vi "PathPlanner_Cmd_AutoHolonomicExecute.vi"(5 "PathPlanner_Cmd_FollowHolConfig":T17={"HOLONOMIC_CTRL_PACK_TUNING"={"X PID Tuning"={"Kp"=0.0, "Ki"=0.0, "Kd"=0.0, "MaximumIntegral"=9.9e+30, "MinimumIntegral"=-9.9e+30, "IntegralZone"=9.9e+30}, "Y PID Tuning"={"Kp"=0.0, "Ki"=0.0, "Kd"=0.0, "MaximumIntegral"=9.9e+30, "MinimumIntegral"=-9.9e+30, "IntegralZone"=9.9e+30}, "thetaProfiledPID_CTRL"={"Controller"={"Kp"=0.0, "Ki"=0.0, "Kd"=0.0, "Period"=0.0, "Max_Integral"=1.0, "Min_Integral"=-1.0, "Max_Input"=0.0, "Min_Input"=0.0, "Continuous"=FALSE, "PositionError"=0.0, "VelocityError"=0.0, "PrevError"=0.0, "Total_Integral"=0.0, "PositionTolerance"=0.05, "VelocityTolerance"=9.99e+35, "SetPoint"=0.0, "Kf"=0.0, "Prev_Deriv"=0.0, "Prev_Deriv 2"=0.0, "DerivativeFilter"=FALSE, "Min_Output"=-9.99e+35, "Max_Output"=9.9e+35, "Prev_F_P"=0.0, "Prev_F_P_2"=0.0, "AntiWindupActive"=FALSE, "Measurement"=0.0, "IntegralZone"=9.9e+30}, "Goal"={"Position"=0.0, "Velocity"=0.0}, "Setpoint"={"Position"=0.0, "Velocity"=0.0}, "Constraint"={"MaxVelocity"=0.0, "MaxAcceleration"=0.0}}}, "Max Wheel Speed M/S"=0.0, "Tolerance SI"={"TRANSLATION"={"X"=0.04, "Y"=0.04}, "ROTATION"={"VALUE"=0.034906585039887, "COS"=0.999390827019096, "SIN"=0.034899496702501}}, "Drive Base Radius M"=0.0, "ControlPastEnd_Sec"=3.0, "Period_Sec"=0.02, "Trigger Events"=TRUE} {"Tolerance SI"."ROTATION"."SIN" format="%13.4f"; "Tolerance SI"."ROTATION"."COS" format="%13.4f"; "Tolerance SI"."ROTATION"."VALUE" format="%13.4f"; "Tolerance SI"."TRANSLATION"."Y" format="%14.3f"; "Tolerance SI"."TRANSLATION"."X" format="%14.3f"; "HOLONOMIC_CTRL_PACK_TUNING"."thetaProfiledPID_CTRL"."Constraint"."MaxAcceleration" format="%16_6e"; "HOLONOMIC_CTRL_PACK_TUNING"."thetaProfiledPID_CTRL"."Constraint"."MaxVelocity" format="%16_6e"; "HOLONOMIC_CTRL_PACK_TUNING"."thetaProfiledPID_CTRL"."Setpoint"."Velocity" format="%16_6e"; "HOLONOMIC_CTRL_PACK_TUNING"."thetaProfiledPID_CTRL"."Setpoint"."Position" format="%16_6e"; "HOLONOMIC_CTRL_PACK_TUNING"."thetaProfiledPID_CTRL"."Goal"."Velocity" format="%16_6e"; "HOLONOMIC_CTRL_PACK_TUNING"."thetaProfiledPID_CTRL"."Goal"."Position" format="%16_6e"; "HOLONOMIC_CTRL_PACK_TUNING"."thetaProfiledPID_CTRL"."Controller"."IntegralZone" format="%16_6e"; "HOLONOMIC_CTRL_PACK_TUNING"."thetaProfiledPID_CTRL"."Controller"."Measurement" format="%16_6e"; "HOLONOMIC_CTRL_PACK_TUNING"."thetaProfiledPID_CTRL"."Controller"."Prev_F_P_2" format="%16_6e"; "HOLONOMIC_CTRL_PACK_TUNING"."thetaProfiledPID_CTRL"."Controller"."Prev_F_P" format="%16_6e"; "HOLONOMIC_CTRL_PACK_TUNING"."thetaProfiledPID_CTRL"."Controller"."Max_Output" format="%16_6e"; "HOLONOMIC_CTRL_PACK_TUNING"."thetaProfiledPID_CTRL"."Controller"."Min_Output" format="%16_6e"; "HOLONOMIC_CTRL_PACK_TUNING"."thetaProfiledPID_CTRL"."Controller"."Prev_Deriv 2" format="%16_6e"; "HOLONOMIC_CTRL_PACK_TUNING"."thetaProfiledPID_CTRL"."Controller"."Prev_Deriv" format="%16_6e"; "HOLONOMIC_CTRL_PACK_TUNING"."thetaProfiledPID_CTRL"."Controller"."Kf" format="%16_6e"; "HOLONOMIC_CTRL_PACK_TUNING"."thetaProfiledPID_CTRL"."Controller"."SetPoint" format="%16_6e"; "HOLONOMIC_CTRL_PACK_TUNING"."thetaProfiledPID_CTRL"."Controller"."VelocityTolerance" format="%16_6e"; "HOLONOMIC_CTRL_PACK_TUNING"."thetaProfiledPID_CTRL"."Controller"."PositionTolerance" format="%16_6e"; "HOLONOMIC_CTRL_PACK_TUNING"."thetaProfiledPID_CTRL"."Controller"."Total_Integral" format="%16_6e"; "HOLONOMIC_CTRL_PACK_TUNING"."thetaProfiledPID_CTRL"."Controller"."PrevError" format="%16_6e"; "HOLONOMIC_CTRL_PACK_TUNING"."thetaProfiledPID_CTRL"."Controller"."VelocityError" format="%16_6e"; "HOLONOMIC_CTRL_PACK_TUNING"."thetaProfiledPID_CTRL"."Controller"."PositionError" format="%16_6e"; "HOLONOMIC_CTRL_PACK_TUNING"."thetaProfiledPID_CTRL"."Controller"."Min_Input" format="%16_6e"; "HOLONOMIC_CTRL_PACK_TUNING"."thetaProfiledPID_CTRL"."Controller"."Max_Input" format="%16_6e"; "HOLONOMIC_CTRL_PACK_TUNING"."thetaProfiledPID_CTRL"."Controller"."Min_Integral" format="%16_6e"; "HOLONOMIC_CTRL_PACK_TUNING"."thetaProfiledPID_CTRL"."Controller"."Max_Integral" format="%16_6e"; "HOLONOMIC_CTRL_PACK_TUNING"."thetaProfiledPID_CTRL"."Controller"."Period" format="%16_6e"; "HOLONOMIC_CTRL_PACK_TUNING"."thetaProfiledPID_CTRL"."Controller"."Kd" format="%16_6e"; "HOLONOMIC_CTRL_PACK_TUNING"."thetaProfiledPID_CTRL"."Controller"."Ki" format="%16_6e"; "HOLONOMIC_CTRL_PACK_TUNING"."thetaProfiledPID_CTRL"."Controller"."Kp" format="%16_6e"}, 6 "PassthroughTime_SEC":dbl=-1.0, 7 "PathPlanner_Cmd_AutoConfig":T2 {"Paths"."IdealStartingState"."Rotation"."SIN" format="%13.4f"; "Paths"."IdealStartingState"."Rotation"."COS" format="%13.4f"; "Paths"."IdealStartingState"."Rotation"."VALUE" format="%13.4f"; "Paths"."PointTowardsZones"."TargetPosition"."Y" format="%14.3f"; "Paths"."PointTowardsZones"."TargetPosition"."X" format="%14.3f"; "Paths"."PointTowardsZones"."RotationOffset"."SIN" format="%13.4f"; "Paths"."PointTowardsZones"."RotationOffset"."COS" format="%13.4f"; "Paths"."PointTowardsZones"."RotationOffset"."VALUE" format="%13.4f"; "Paths"."Waypoints"."nextControl"."Y" format="%14.3f"; "Paths"."Waypoints"."nextControl"."X" format="%14.3f"; "Paths"."Waypoints"."anchor"."Y" format="%14.3f"; "Paths"."Waypoints"."anchor"."X" format="%14.3f"; "Paths"."Waypoints"."prevControl"."Y" format="%14.3f"; "Paths"."Waypoints"."prevControl"."X" format="%14.3f"; "Paths"."AllPoints"."RotationTarget"."rotation"."SIN" format="%13.4f"; "Paths"."AllPoints"."RotationTarget"."rotation"."COS" format="%13.4f"; "Paths"."AllPoints"."RotationTarget"."rotation"."VALUE" format="%13.4f"; "Paths"."AllPoints"."Position"."Y" format="%14.3f"; "Paths"."AllPoints"."Position"."X" format="%14.3f"; "Paths"."GoalEndState"."Rotation"."SIN" format="%13.4f"; "Paths"."GoalEndState"."Rotation"."COS" format="%13.4f"; "Paths"."GoalEndState"."Rotation"."VALUE" format="%13.4f"; "Paths"."RotationTargets"."rotation"."SIN" format="%13.4f"; "Paths"."RotationTargets"."rotation"."COS" format="%13.4f"; "Paths"."RotationTargets"."rotation"."VALUE" format="%13.4f"}, 8 "Enabled":bool=TRUE, 9 "Reset":bool, 10 "CurrentChassisSpeeds":T1 {"vOmega" format="%10.3f"; "vY" format="%10.3f"; "vX" format="%10.3f"}, 11 "Current Pose SI":T24={"TRANSLATION"={"X"=0.0, "Y"=0.0}, "ROTATION"={"VALUE"=0.0, "COS"=1.0, "SIN"=0.0}} {"ROTATION"."SIN" format="%13.4f"; "ROTATION"."COS" format="%13.4f"; "ROTATION"."VALUE" format="%13.4f"; "TRANSLATION"."Y" format="%14.3f"; "TRANSLATION"."X" format="%14.3f"}) -> (0 "Position Error M":dbl, 1 "Complete":bool, 2 "At Reference":bool, 3 "calcChassisSpeed":T1 {"vOmega" format="%10.3f"; "vY" format="%10.3f"; "vX" format="%10.3f"})   [LabVIEW 2019, in "PathPlanner24.lvlib"]
doc: "DOCUMENTATION IS NOT COMPLETE.\n \nCalculates the next output of the path following controller for holonomic drive robots. This wraps a Holonomic Drive Control function with the particulars needed to follow a PathPlanner trajectory.\n\nInputs:\n - PathPlanner_Holonomic_Ctrl_Pack_Tuning - cluster - The tuning paraameters for the holonomic drive controller. These are static. They should not be changed after the first call to this function.\n - CurrentPoseSi - pose2d - The current pose calculated by odometry or pose estimation. The pose can be absolute or relative depending on what type of trajectory is being followed.\n - PathPlannerState - cluster - The path palnner trajectory state containing the desired position and velocities of the robot.\n - Reset - boolean - When TRUE the holonomic drive controller is reset. This should be set to TRUE for the first execution of a trajectory.\n - Enabled - boolean - When TRUE, closed loop control is enabled. (Optional. Default: TRUE)\n - Period - double - The loop period in seconds for this controller. (Optional. Default: 0.020)\n\nOutputs:\n - CalcChassisSpeed - cluster - The desired chassis speed in SI units.\n - AtReference - boolean - TRUE if the robots position is within the defined tolerance.\n - PositionError - pose2d - Position error in SI units. How far the robot is away from the desired trajectory position.\n - out_Holonomic_Drive_Ctrl - THe current holonomic drive controller data cluster. This is mainly for diagnostic purposes."
uses:
  PathPlanner24.lvlib
  <vilib>/Rock Robotics/WPI/ThirdParty/JAS_Junk/TrajLib/Trajectory_Library.lvlib
  <vilib>/Rock Robotics/WPI/ThirdParty/JAS_Junk/TrajLib/TypeDef/CHASSIS_SPEEDS.ctl
  <vilib>/Rock Robotics/WPI/ThirdParty/JAS_Junk/TrajLib/TypeDef/TRANSLATION2D.ctl
  <vilib>/Rock Robotics/WPI/ThirdParty/JAS_Junk/TrajLib/TypeDef/ROTATION2D.ctl
  <vilib>/Rock Robotics/WPI/ThirdParty/JAS_Junk/TrajLib/TypeDef/POSE2D.ctl
  <vilib>/Rock Robotics/WPI/ThirdParty/JAS_Junk/TrajLib/TypeDef/PID_TUNING.ctl
  <vilib>/Rock Robotics/WPI/ThirdParty/JAS_Junk/TrajLib/TypeDef/PID_CONTROLLER.ctl
  <vilib>/Rock Robotics/WPI/ThirdParty/JAS_Junk/TrajLib/TypeDef/TRAPEZOID_PROFILE_STATE.ctl
  <vilib>/Rock Robotics/WPI/ThirdParty/JAS_Junk/TrajLib/TypeDef/TRAPEZOID_PROFILE_CONSTRAINT.ctl
  <vilib>/Rock Robotics/WPI/ThirdParty/JAS_Junk/TrajLib/TypeDef/PROFILED_PID_CONTROLLER.ctl
  <vilib>/Rock Robotics/WPI/ThirdParty/JAS_Junk/TrajLib/TypeDef/HOLONOMIC_PACK_TUNING.ctl
  TypeDef/PathPlannerRotationTarget.ctl
  TypeDef/PathPlannerPathConstraints.ctl
  TypeDef/PathPlannerConstraintsZone.ctl
  ENum/PathPlanner_CommandUtilType_ENUM.ctl
  TypeDef/PathPlannerCommandUtil.ctl
  TypeDef/PathPlannerEventMarker.ctl
  TypeDef/PathPlannerGoalEndState.ctl
  TypeDef/PathPlannerPathPoint.ctl
  TypeDef/PathPlannerPath.ctl
  TypeDef/PathPlannerCmdFollowHolConfig.ctl
  TypeDef/PathPlannerWaypoint.ctl
  TypeDef/PathPlannerPointTowardsZone.ctl
  TypeDef/PathPlannerIdealStartingState.ctl
  TypeDef/PathPlannerCmdPathPlannerAutoConfig.ctl
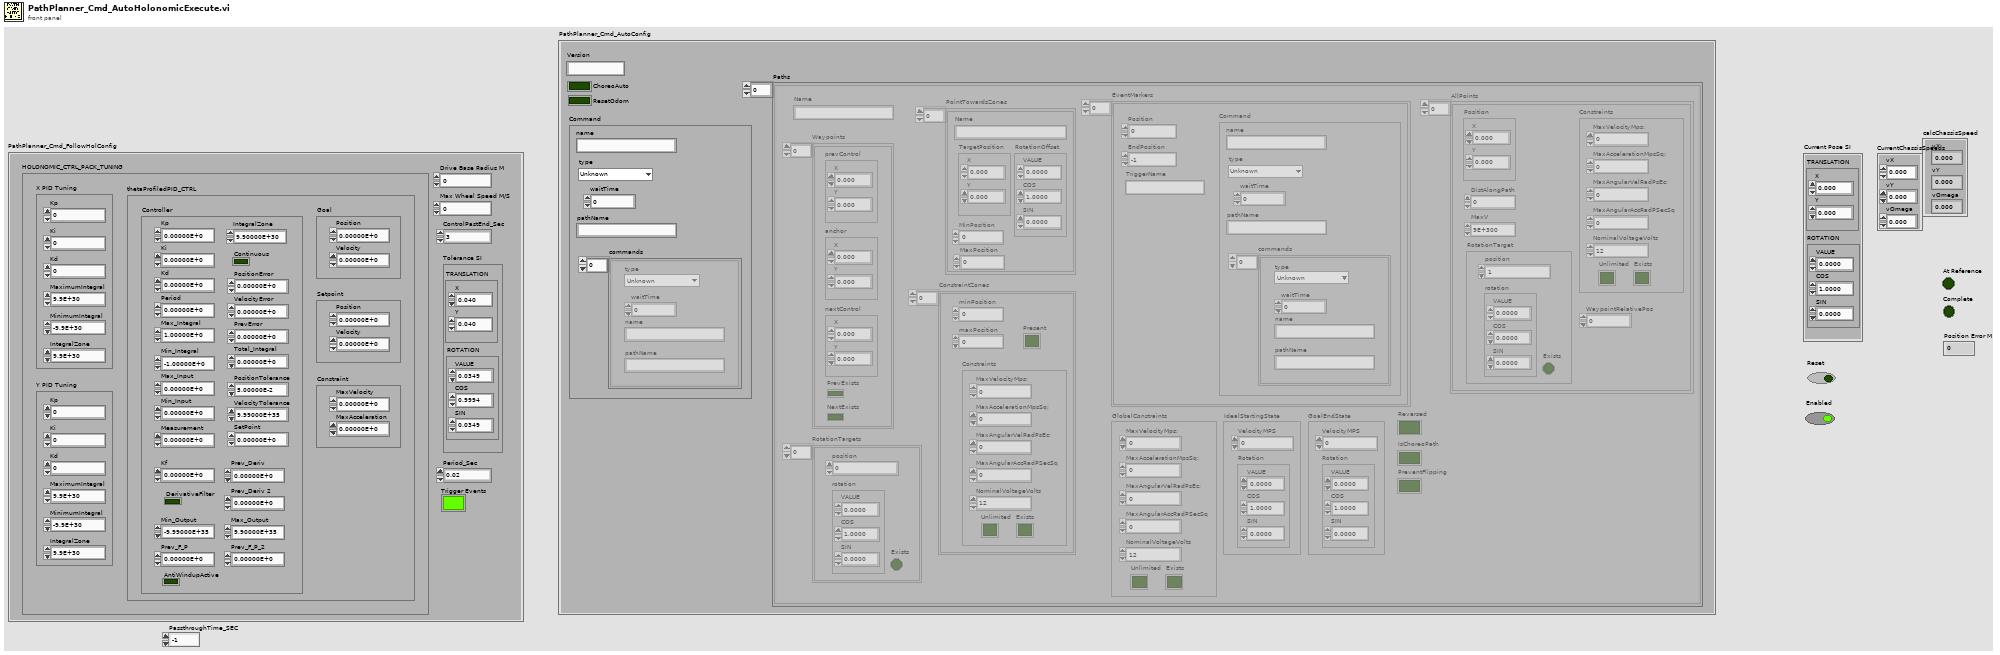
[diagram p1: front panel]
types:
  T1 = typedef "Trajectory_Library.lvlib/CHASSIS_SPEEDS.ctl" = cluster{"vX":dbl, "vY":dbl, "vOmega":dbl}
  T2 = typedef "PathPlanner24.lvlib/PathPlannerCmdPathPlannerAutoConfig.ctl" = cluster{"Command":T3, "ChoreoAuto":bool, "Version":string, "ResetOdom":bool, "Paths":T5[]}
  T3 = typedef "PathPlanner24.lvlib/PathPlannerCommandUtil.ctl" = cluster{"waitTime":dbl, "name":string, "pathName":string, "commands":cluster{"type":T4, "waitTime":dbl, "name":string, "pathName":string}[], "type":T4}
  T4 = typedef "PathPlanner24.lvlib/PathPlanner_CommandUtilType_ENUM.ctl" = enum16{"Unknown", "Wait", "Named", "Path", "Sequential", "Parallel", "Race", "Deadline"}
  T5 = typedef "PathPlanner24.lvlib/PathPlannerPath.ctl" = cluster{"Reversed":bool, "RotationTargets":T6[], "ConstraintZones":T8[], "EventMarkers":T10[], "GlobalConstraints":T9, "GoalEndState":T11, "AllPoints":T12[], "Name":string, "Waypoints":T14[], "PointTowardsZones":T15[], "IdealStartingState":T16, "IsChoreoPath":bool, "PreventFlipping":bool}
  T6 = typedef "PathPlanner24.lvlib/PathPlannerRotationTarget.ctl" = cluster{"position":dbl, "rotation":T7, "Exists":bool}
  T7 = typedef "Trajectory_Library.lvlib/ROTATION2D.ctl" = cluster{"VALUE":dbl, "COS":dbl, "SIN":dbl}
  T8 = typedef "PathPlanner24.lvlib/PathPlannerConstraintsZone.ctl" = cluster{"minPosition":dbl, "maxPosition":dbl, "Constraints":T9, "Present":bool}
  T9 = typedef "PathPlanner24.lvlib/PathPlannerPathConstraints.ctl" = cluster{"MaxVelocityMps;":dbl, "MaxAccelerationMpsSq;":dbl, "MaxAngularVelRadPsEc;":dbl, "MaxAngularAccRadPSecSq":dbl, "Exists":bool, "Unlimited":bool, "NominalVoltageVolts":dbl}
  T10 = typedef "PathPlanner24.lvlib/PathPlannerEventMarker.ctl" = cluster{"Position":dbl, "Command":T3, "TriggerName":string, "EndPosition":dbl}
  T11 = typedef "PathPlanner24.lvlib/PathPlannerGoalEndState.ctl" = cluster{"VelocityMPS":dbl, "Rotation":T7}
  T12 = typedef "PathPlanner24.lvlib/PathPlannerPathPoint.ctl" = cluster{"Position":T13, "DistAlongPath":dbl, "MaxV":dbl, "Constraints":T9, "RotationTarget":T6, "WaypointRelativePos":dbl}
  T13 = typedef "Trajectory_Library.lvlib/TRANSLATION2D.ctl" = cluster{"X":dbl, "Y":dbl}
  T14 = typedef "PathPlanner24.lvlib/PathPlannerWaypoint.ctl" = cluster{"prevControl":T13, "anchor":T13, "nextControl":T13, "PrevExists":bool, "NextExists":bool}
  T15 = typedef "PathPlanner24.lvlib/PathPlannerPointTowardsZone.ctl" = cluster{"RotationOffset":T7, "Name":string, "TargetPosition":T13, "MinPosition":dbl, "MaxPosition":dbl}
  T16 = typedef "PathPlanner24.lvlib/PathPlannerIdealStartingState.ctl" = cluster{"VelocityMPS":dbl, "Rotation":T7}
  T17 = typedef "PathPlanner24.lvlib/PathPlannerCmdFollowHolConfig.ctl" = cluster{"HOLONOMIC_CTRL_PACK_TUNING":T18, "Max Wheel Speed M/S":dbl, "Tolerance SI":T24, "Drive Base Radius M":dbl, "ControlPastEnd_Sec":dbl, "Period_Sec":dbl, "Trigger Events":bool}
  T18 = typedef "Trajectory_Library.lvlib/HOLONOMIC_PACK_TUNING.ctl" = cluster{"X PID Tuning":T19, "Y PID Tuning":T19, "thetaProfiledPID_CTRL":T20}
  T19 = typedef "Trajectory_Library.lvlib/PID_TUNING.ctl" = cluster{"Kp":dbl, "Ki":dbl, "Kd":dbl, "MaximumIntegral":dbl, "MinimumIntegral":dbl, "IntegralZone":dbl}
  T20 = typedef "Trajectory_Library.lvlib/PROFILED_PID_CONTROLLER.ctl" = cluster{"Controller":T21, "Goal":T22, "Setpoint":T22, "Constraint":T23}
  T21 = typedef "Trajectory_Library.lvlib/PID_CONTROLLER.ctl" = cluster{"Kp":dbl, "Ki":dbl, "Kd":dbl, "Period":dbl, "Max_Integral":dbl, "Min_Integral":dbl, "Max_Input":dbl, "Min_Input":dbl, "Continuous":bool, "PositionError":dbl, "VelocityError":dbl, "PrevError":dbl, "Total_Integral":dbl, "PositionTolerance":dbl, "VelocityTolerance":dbl, "SetPoint":dbl, "Kf":dbl, "Prev_Deriv":dbl, "Prev_Deriv 2":dbl, "DerivativeFilter":bool, "Min_Output":dbl, "Max_Output":dbl, "Prev_F_P":dbl, "Prev_F_P_2":dbl, "AntiWindupActive":bool, "Measurement":dbl, "IntegralZone":dbl}
  T22 = typedef "Trajectory_Library.lvlib/TRAPEZOID_PROFILE_STATE.ctl" = cluster{"Position":dbl, "Velocity":dbl}
  T23 = typedef "Trajectory_Library.lvlib/TRAPEZOID_PROFILE_CONSTRAINT.ctl" = cluster{"MaxVelocity":dbl, "MaxAcceleration":dbl}
  T24 = typedef "Trajectory_Library.lvlib/POSE2D.ctl" = cluster{"TRANSLATION":T13, "ROTATION":T7}
  T25 = typedef "Trajectory_Library.lvlib/TIMER.ctl" = cluster{"StartTime":dbl, "Accumulated TIme":dbl, "Running":bool, "semaphore":T26}
  T26 = typedef "Semaphore RefNum" = refnum<k1>
  T27 = cluster{"type":T4, "waitTime":dbl, "name":string, "pathName":string}[]
  T28 = cluster{"type":T4, "waitTime":dbl, "name":string, "pathName":string}
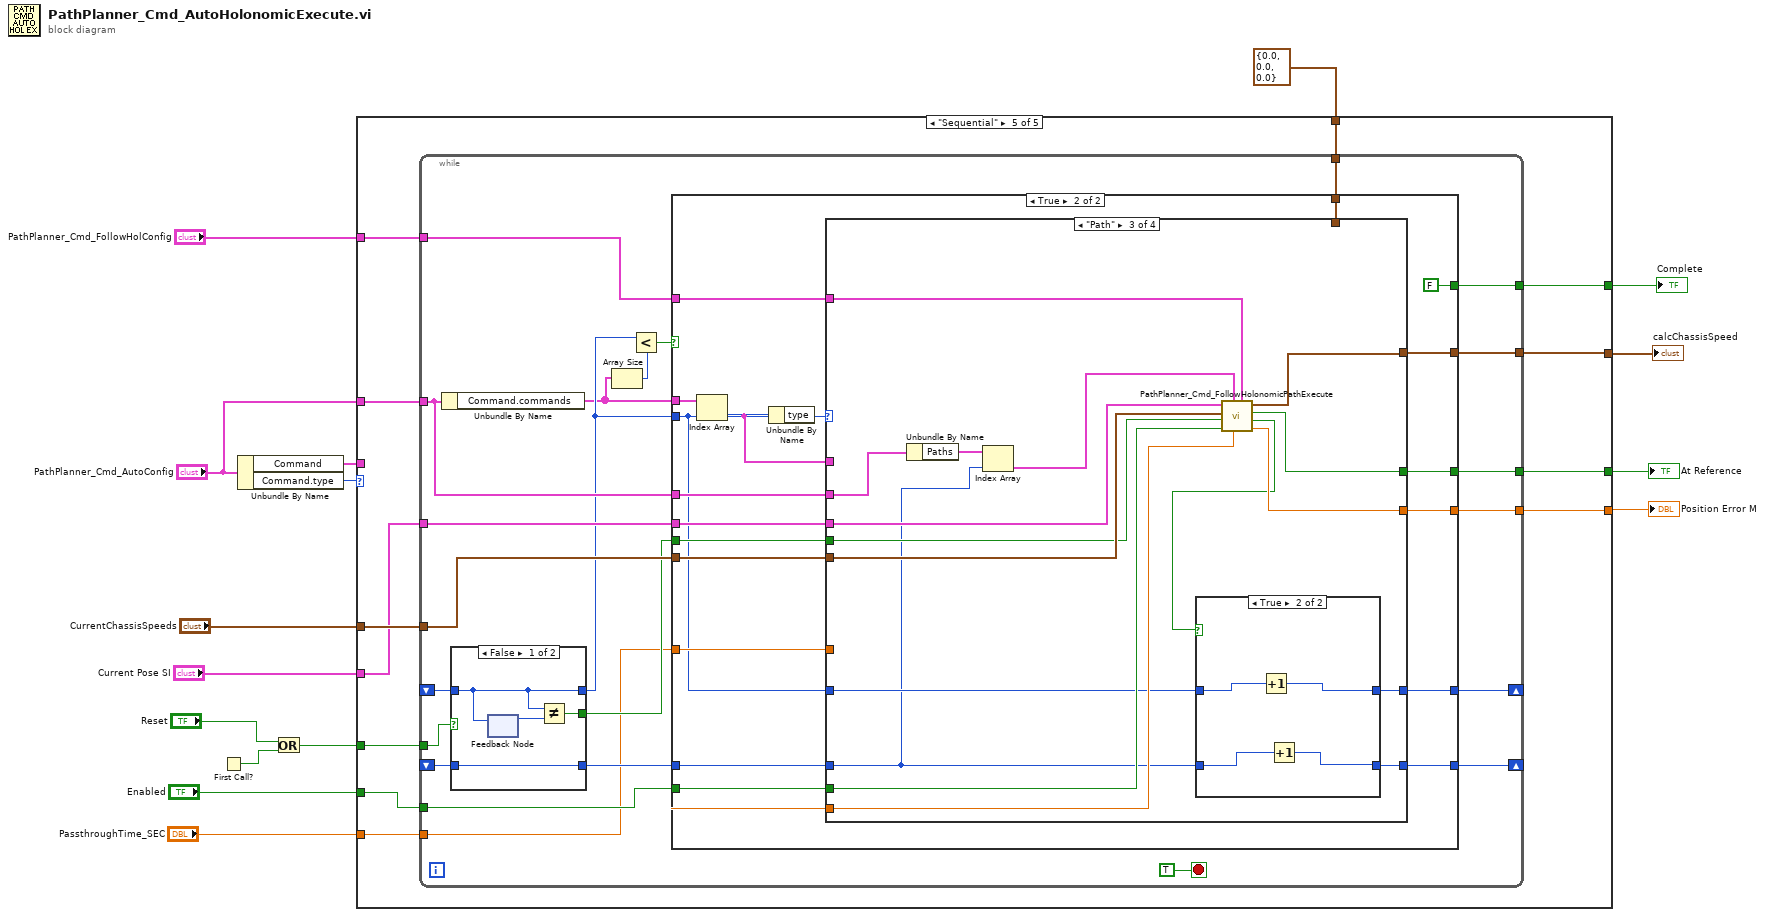
[diagram p0: block diagram]
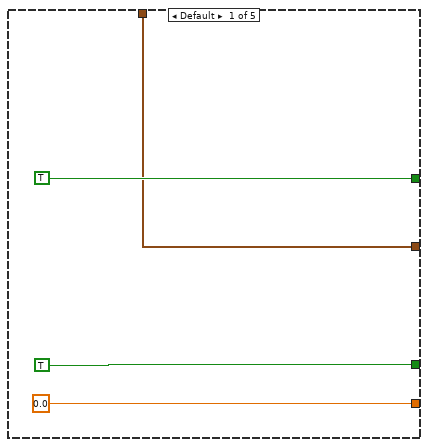
[diagram p2: hidden frame]
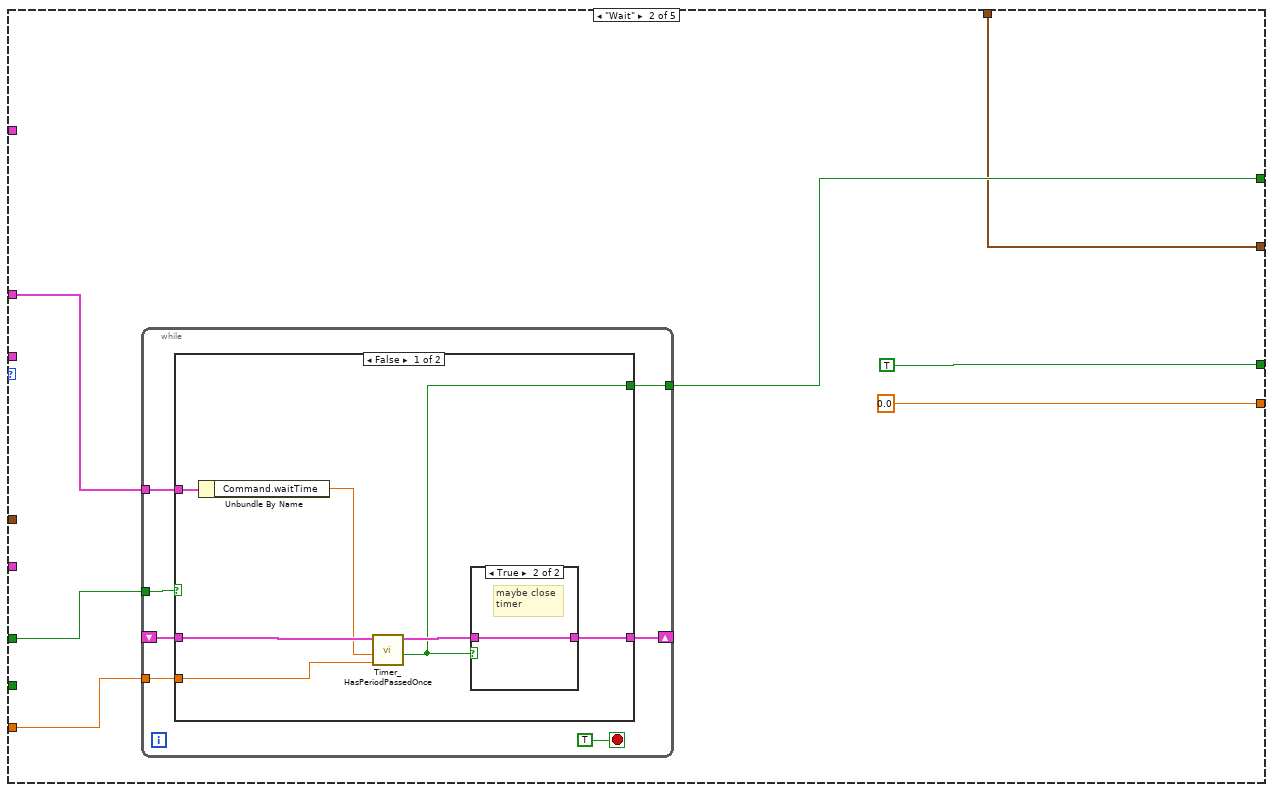
[diagram p3: hidden frame]
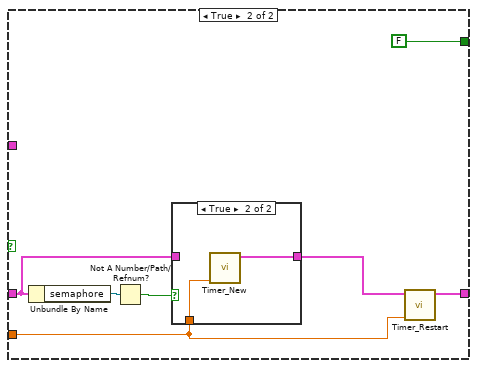
[diagram p5: hidden frame]
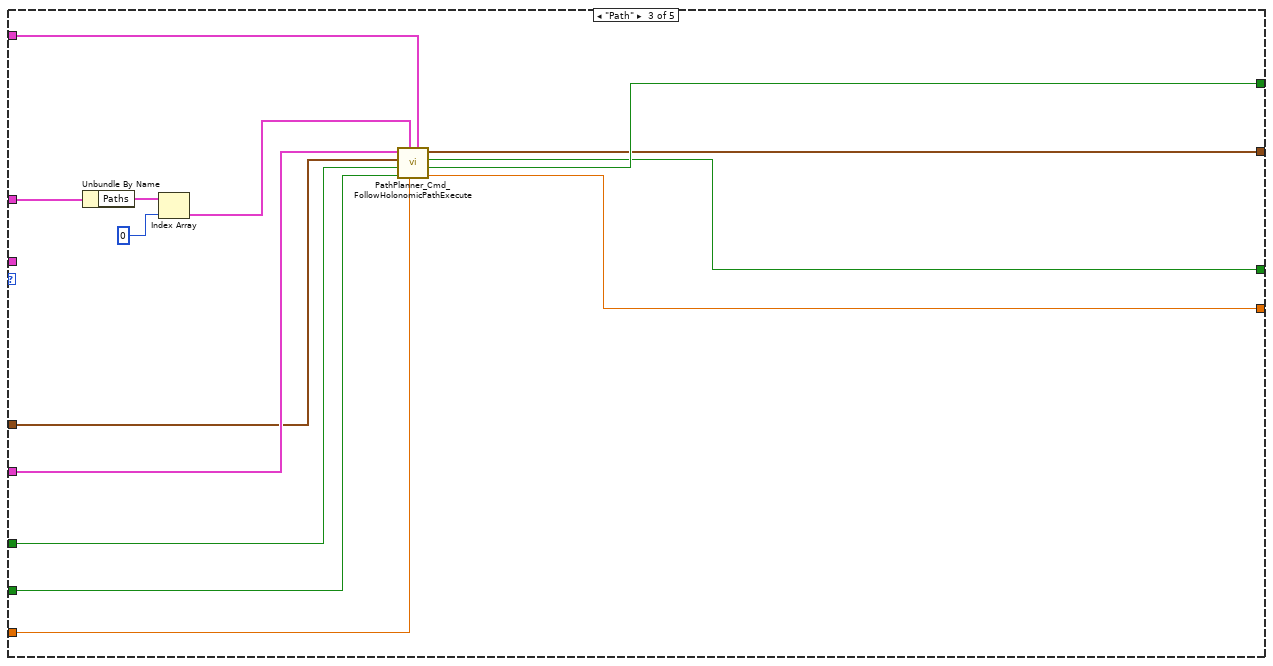
[diagram p7: hidden frame]
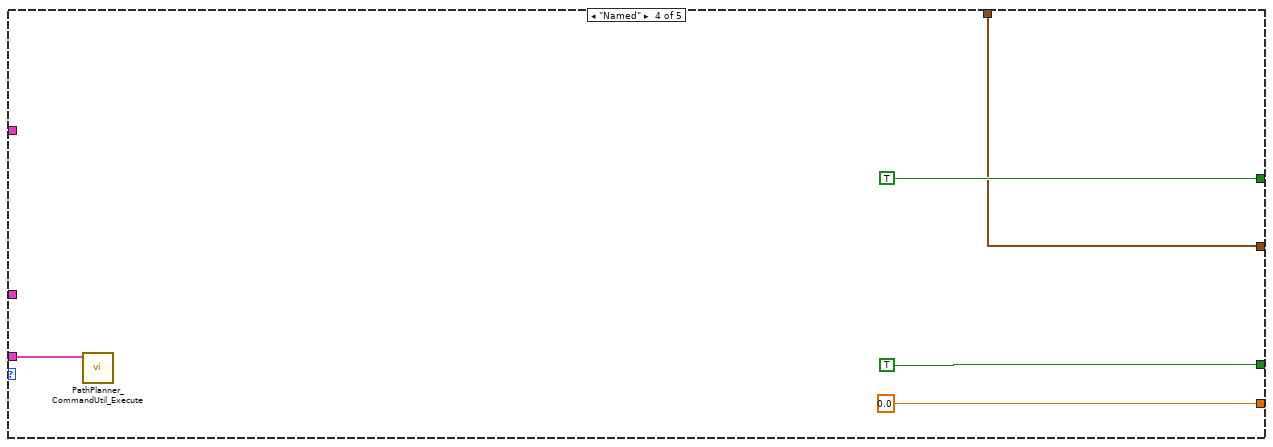
[diagram p8: hidden frame]
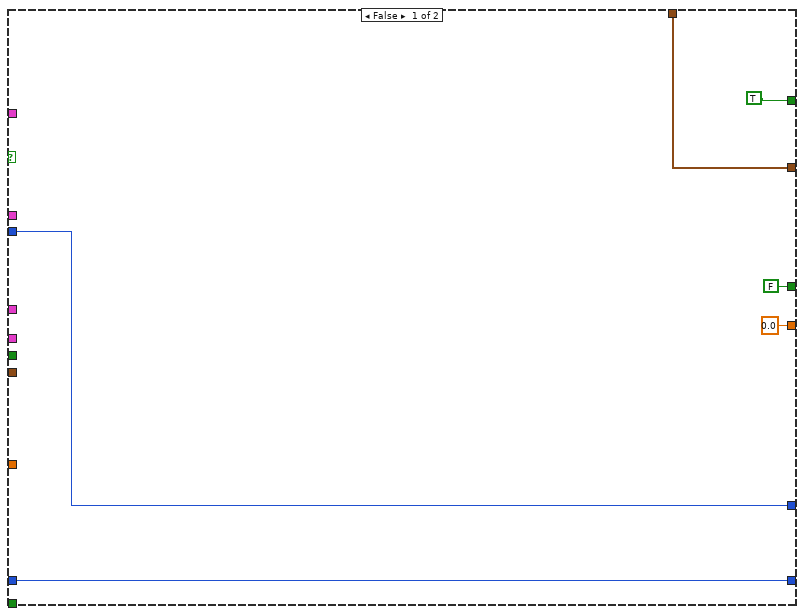
[diagram p9: hidden frame]
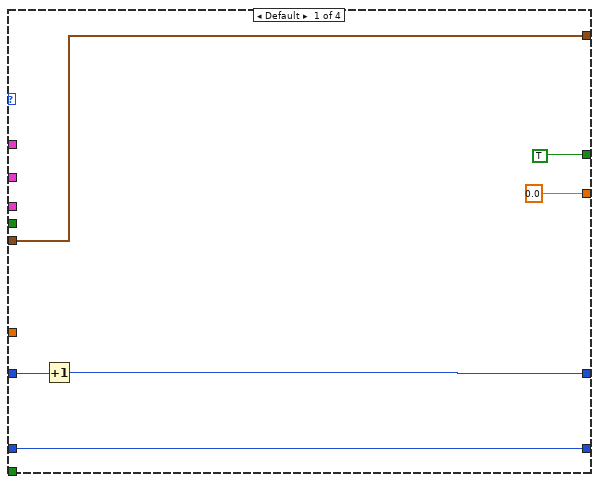
[diagram p10: hidden frame]
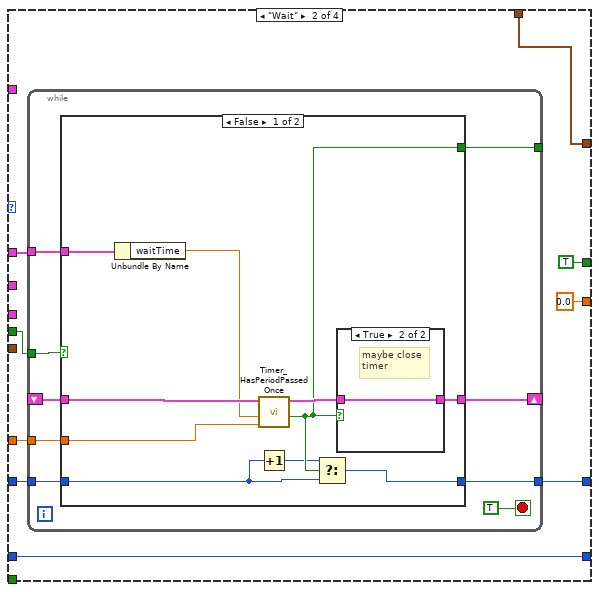
[diagram p11: hidden frame]
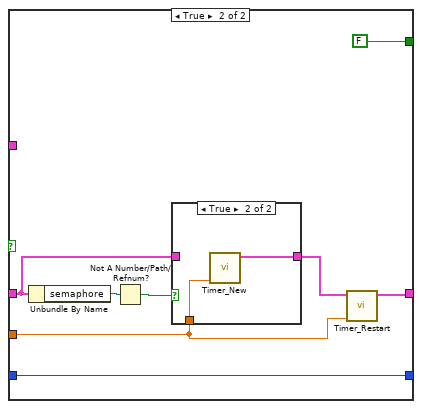
[diagram p13: hidden frame]
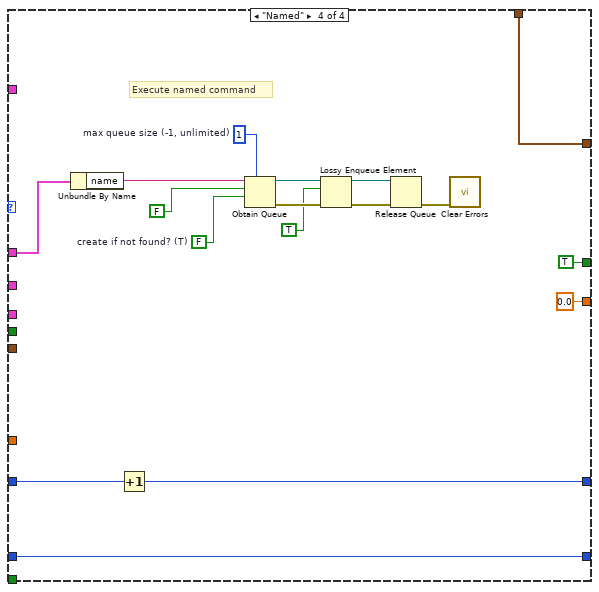
[diagram p16: hidden frame]
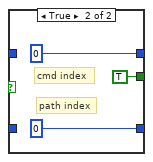
[diagram p17: hidden frame]
diagram:
  n1 = First Call?() -> (First Call?: T/F=w15:bool)
  n2 = Unbundle By Name("PathPlanner_Cmd_AutoConfig") -> ("Command"=w13:T3, "Command.type"=w14:T4)
  n3 = Or(x="Reset", y=w15) -> (x .or. y?=w8:bool)
  n4 = case shown="\"Sequential\"" w14 {
    tunnel: w13 -> [_ _ _ w72 _]
    tunnel: "PathPlanner_Cmd_AutoConfig" -> [_ w25 w67 _ w83]
    tunnel: "PathPlanner_Cmd_FollowHolConfig" -> [_ _ w63 _ w76]
    tunnel: "Current Pose SI" -> [_ _ w62 _ w75]
    tunnel: "CurrentChassisSpeeds" -> [_ _ w61 _ w82]
    tunnel: w8 -> [_ w27 w60 _ w84]
    tunnel: "Enabled" -> [_ _ w59 _ w74]
    tunnel: "PassthroughTime_SEC" -> [_ w26 w58 _ w78]
    tunnel: [0.0 ("Position Error M") 0.0 ("Position Error M") w57 0.0 ("Position Error M") w79] -> w5
    tunnel: [TRUE ("Complete") w24 w56 TRUE ("Complete") w73] -> w4
    tunnel: [TRUE ("At Reference") TRUE ("At Reference") w55 TRUE ("At Reference") w80] -> w3
    tunnel: [w17 w21 w54 w68 w81] -> w2
    tunnel: T1 {"vX"=0.0, "vY"=0.0, "vOmega"=0.0} ("CurrentChassisSpeeds") -> [w17 w21 _ w68 w77]
    frame Default {
    }
    frame "Wait" {
      n5 = while {
        tunnel: w27 -> [w34]
        tunnel: w26 -> [w33]
        shift-right: [w32] -> _
        shift-left: _ -> [w31]
        tunnel: w25 -> [w30]
        tunnel: [w28] -> w24
        stop <- TRUE stop-if-true
        n6 = case shown="False" w34 {
          tunnel: w33 -> [w40 w49]
          tunnel: [w36 w48] -> w32
          tunnel: w31 -> [w41 w44]
          tunnel: w30 -> [w39 _]
          tunnel: [w35 FALSE ("Expired")] -> w28
          frame False {
            n7 = Unbundle By Name(w39) -> ("Command.waitTime"=w38:dbl)
            n8 = call <vilib>:"Timer_HasPeriodPassedOnce.vi"("Pass_Through_Time"=w40, "Period"=w38, "in Timer"=w41) -> ("Expired"=w35:bool, "out Timer"=w37:T25)  [unwired: 6 in, 1 out]
            n9 = case shown="True" w35 {
              tunnel: w37 -> [w42 w43]
              tunnel: [w42 w43] -> w36
              frame False {
              }
              frame True {
                # "maybe close\ntimer"
              }
            }
          }
          frame True {
            n10 = Unbundle By Name(w44) -> ("semaphore"=w45:T26)
            n11 = Not A Number/Path/Refnum?(number/path/refnum=w45) -> (NaN/Path/Refnum?=w46:bool)
            n12 = case shown="True" w46 {
              tunnel: [w51 w53] -> w50
              tunnel: w49 -> [_ w52]
              tunnel: w44 -> [w51 _]
              frame False {
              }
              frame True {
                n13 = call <vilib>:"Timer_New.vi"("Pass_Through_Time"=w52) -> ("TIMER"=w53:T25)  [unwired: 10 in]
              }
            }
            n14 = call <vilib>:"Timer_Restart.vi"("Pass_Through_Time"=w49, "in Timer"=w50) -> ("out Timer"=w48:T25)  [unwired: 9 in]
          }
        }
      }
    }
    frame "Path" {
      n15 = Unbundle By Name(w67) -> ("Paths"=w66:T5[])
      n16 = Index Array(array=w66, index=0) -> (element=w64:T5)
      n17 = call "PathPlanner_Cmd_FollowHolonomicPathExecute.vi"("PathPlanner_Cmd_FollowHolConfig"=w63, "PassthroughTime_SEC"=w58, "PathPlannerPath"=w64, "Enabled"=w59, "Reset"=w60, "CurrentChassisSpeeds"=w61, "Current Pose SI"=w62) -> ("Position Error M"=w57:dbl, "Complete"=w56:bool, "At Reference"=w55:bool, "calcChassisSpeed"=w54:T1)  [unwired: 1 out]
    }
    frame "Named" {
      n18 = call "PathPlanner_CommandUtil_Execute.vi"("Command"=w72) -> ()  [unwired: 11 in]
    }
    frame "Sequential" {
      n19 = while {
        tunnel: w84 -> [w102]
        tunnel: w83 -> [w97]
        tunnel: w82 -> [w106]
        tunnel: [w105] -> w81
        tunnel: [w104] -> w80
        tunnel: [w103] -> w79
        tunnel: w78 -> [w92]
        shift-right: [w91] -> _
        shift-left: _ -> [w101]
        shift-right: [w90] -> _
        shift-left: _ -> [w100]
        tunnel: w77 -> [w98]
        tunnel: w76 -> [w95]
        tunnel: w75 -> [w94]
        tunnel: w74 -> [w93]
        tunnel: [w85] -> w73
        stop <- TRUE stop-if-true
        n20 = Unbundle By Name(w97) -> ("Command.commands"=w87:T27)
        n21 = case shown="False" w102 {
          tunnel: [w220 0] -> w89
          tunnel: [w222 0] -> w96
          tunnel: w101 -> [w220 _]
          tunnel: w100 -> [w222 _]
          tunnel: [w223 TRUE] -> w99
          frame False {
            n22 = feedback-in #1(w220) -> ()
            n23 = feedback #1() -> (w221:i32)  [unwired: 1 in]
            n24 = Not Equal?(x=w220, y=w221) -> (x != y?=w223:bool)
          }
          frame True {
            # "path index"
            # "cmd index"
          }
        }
        n25 = Array Size(array=w87) -> (size(s)=w88:i32)
        n26 = Less?(x=w89, y=w88) -> (x < y?=w86:bool)
        n27 = case shown="True" w86 {
          tunnel: w106 -> [_ w132]
          tunnel: [w112 w131] -> w105
          tunnel: [FALSE ("At Reference") w130] -> w104
          tunnel: [0.0 ("Position Error M") w129] -> w103
          tunnel: w87 -> [_ w128]
          tunnel: w99 -> [_ w126]
          tunnel: w98 -> [w112 w124]
          tunnel: w97 -> [_ w123]
          tunnel: w96 -> [w108 w122]
          tunnel: w95 -> [_ w121]
          tunnel: w94 -> [_ w120]
          tunnel: w93 -> [_ w119]
          tunnel: w92 -> [_ w118]
          tunnel: w89 -> [w109 w114]
          tunnel: [w109 w117] -> w91
          tunnel: [w108 w116] -> w90
          tunnel: [TRUE FALSE] -> w85
          frame False {
          }
          frame True {
            n28 = Index Array(array=w128, index=w114) -> (element=w125:T28)
            n29 = Unbundle By Name(w125) -> ("type"=w127:T4)
            n30 = case shown="\"Path\"" w127 {
              tunnel: w132 -> [w138 _ w191 _]
              tunnel: [w138 w144 w187 w208] -> w131
              tunnel: [TRUE TRUE ("At Reference") w186 TRUE ("At Reference")] -> w130
              tunnel: [0.0 0.0 ("Position Error M") w185 0.0 ("Position Error M")] -> w129
              tunnel: w118 -> [_ w147 _ _]
              tunnel: w126 -> [_ w146 w190 _]
              tunnel: w125 -> [_ w145 _ w209]
              tunnel: w124 -> [_ w144 _ w208]
              tunnel: w123 -> [_ _ w194 _]
              tunnel: w122 -> [w133 w143 w182 w203]
              tunnel: w121 -> [_ _ w193 _]
              tunnel: w120 -> [_ _ w192 _]
              tunnel: w119 -> [_ _ w189 _]
              tunnel: w118 -> [_ _ w188 _]
              tunnel: w114 -> [w135 w142 w183 w205]
              tunnel: [w134 w141 w180 w204] -> w117
              tunnel: [w133 w143 w181 w203] -> w116
              frame Default {
                n31 = Increment(x=w135) -> (x+1=w134:i32)
              }
              frame "Wait" {
                n32 = while {
                  tunnel: w146 -> [w156]
                  tunnel: w147 -> [w155]
                  shift-right: [w154] -> _
                  shift-left: _ -> [w153]
                  tunnel: w145 -> [w152]
                  tunnel: [w150] -> _
                  tunnel: w142 -> [w149]
                  tunnel: [w148] -> w141
                  stop <- TRUE stop-if-true
                  n33 = case shown="False" w156 {
                    tunnel: w155 -> [w165 w175]
                    tunnel: [w161 w174] -> w154
                    tunnel: w153 -> [w166 w170]
                    tunnel: w152 -> [w164 _]
                    tunnel: [w160 FALSE ("Expired")] -> w150
                    tunnel: w149 -> [w157 w169]
                    tunnel: [w159 w169] -> w148
                    frame False {
                      n34 = Unbundle By Name(w164) -> ("waitTime"=w163:dbl)
                      n35 = call <vilib>:"Timer_HasPeriodPassedOnce.vi"("Pass_Through_Time"=w165, "Period"=w163, "in Timer"=w166) -> ("Expired"=w160:bool, "out Timer"=w162:T25)  [unwired: 6 in, 1 out]
                      n36 = Increment(x=w157) -> (x+1=w158:i32)
                      n37 = Select(t=w158, s=w160, f=w157) -> (s? t:f=w159:i32)
                      n38 = case shown="True" w160 {
                        tunnel: w162 -> [w167 w168]
                        tunnel: [w167 w168] -> w161
                        frame False {
                        }
                        frame True {
                          # "maybe close\ntimer"
                        }
                      }
                    }
                    frame True {
                      n39 = Unbundle By Name(w170) -> ("semaphore"=w171:T26)
                      n40 = Not A Number/Path/Refnum?(number/path/refnum=w171) -> (NaN/Path/Refnum?=w172:bool)
                      n41 = case shown="True" w172 {
                        tunnel: [w177 w179] -> w176
                        tunnel: w175 -> [_ w178]
                        tunnel: w170 -> [w177 _]
                        frame False {
                        }
                        frame True {
                          n42 = call <vilib>:"Timer_New.vi"("Pass_Through_Time"=w178) -> ("TIMER"=w179:T25)  [unwired: 10 in]
                        }
                      }
                      n43 = call <vilib>:"Timer_Restart.vi"("Pass_Through_Time"=w175, "in Timer"=w176) -> ("out Timer"=w174:T25)  [unwired: 9 in]
                    }
                  }
                }
              }
              frame "Path" {
                n44 = Unbundle By Name(w194) -> ("Paths"=w196:T5[])
                n45 = Index Array(array=w196, index=w182) -> (element=w195:T5)
                n46 = call "PathPlanner_Cmd_FollowHolonomicPathExecute.vi"("PathPlanner_Cmd_FollowHolConfig"=w193, "PassthroughTime_SEC"=w188, "PathPlannerPath"=w195, "Enabled"=w189, "Reset"=w190, "CurrentChassisSpeeds"=w191, "Current Pose SI"=w192) -> ("Position Error M"=w185:dbl, "Complete"=w184:bool, "At Reference"=w186:bool, "calcChassisSpeed"=w187:T1)  [unwired: 1 out]
                n47 = case shown="True" w184 {
                  tunnel: w183 -> [w197 w202]
                  tunnel: w182 -> [w198 w200]
                  tunnel: [w198 w199] -> w181
                  tunnel: [w197 w201] -> w180
                  frame False {
                  }
                  frame True {
                    n48 = Increment(x=w202) -> (x+1=w201:i32)
                    n49 = Increment(x=w200) -> (x+1=w199:i32)
                  }
                }
              }
              frame "Named" {
                w215 = FALSE  # create if not found? (T)
                w214 = 1  # max queue size (-1, unlimited)
                # "Execute named command"
                n50 = Unbundle By Name(w209) -> ("name"=w213:string)
                n51 = Increment(x=w205) -> (x+1=w204:i32)
                n52 = Obtain Queue(max queue size (-1, unlimited)=w214, name (unnamed)=w213, element data type=FALSE, create if not found? (T)=w215) -> (queue out=w218:refnum<queue>, error out=w219:errorcluster)  [unwired: 1 in, 1 out]
                n53 = Lossy Enqueue Element(queue=w218, element=TRUE, error in (no error)=w219) -> (queue out=w210:refnum<queue>, error out=w211:errorcluster)  [unwired: 2 out]
                n54 = Release Queue(queue=w210, error in (no error)=w211) -> (error out=w212:errorcluster)  [unwired: 1 in, 2 out]
                n55 = call <vilib>:"Clear Errors.vi"("error in (no error)"=w212) -> ()  [unwired: 5 in, 2 out]
              }
            }
          }
        }
      }
    }
  }
  "At Reference" <- w3
  "Position Error M" <- w5
  "calcChassisSpeed" <- w2
  "Complete" <- w4
